vi "Stop Core.vi"(10 "final error code":i32, 11 "DAQMan in":refnum<class "Cfg Grandmaster.lvclass">) -> (3 "DAQMan out":refnum<class "Cfg Grandmaster.lvclass">)   [LabVIEW 2018, in "Configuration Grandmaster.lvlib" / "Cfg Grandmaster.lvclass"]
doc: "(<B>Filename</B>: Actor Framework.lvlib:Actor.lvclass:Stop Core.vi)\n\nDefines what the actor does before it stops. Use the <B>final error code</B> input to determine whether the actor shut down in response to an error.\n\nBy default, this method does nothing. A descendant class may override it to define behavior, such as shutting down any processes the actor initiated in its override of the Actor Core method."
uses:
  Cfg Grandmaster.lvclass
  Cfg Grandmaster.lvclass/Cfg Grandmaster.ctl
  <vilib>/ActorFramework/Stop Msg/Stop Msg.lvclass/Stop Msg.ctl
  <vilib>/ActorFramework/Message Enqueuer/Message Enqueuer.lvclass/Message Enqueuer.ctl
  <vilib>/ActorFramework/Stop Msg/Send Emergency Stop.vi
  <vilib>/ActorFramework/Stop Msg/Send Normal Stop.vi
  <vilib>/ActorFramework/Message Enqueuer/Enqueue Critical.vi
  <vilib>/ActorFramework/Message Enqueuer/Enqueue.vi
  <vilib>/ActorFramework/Stop Msg/Stop Msg.lvclass
  C:/Program Files (x86)/National Instruments/LabVIEW 2018/vi.lib/ActorFramework/Message/Message.lvclass
  <vilib>/ActorFramework/Message Priority Queue/Priority Enqueue.vi
  Actor Nest/Class Actor Nest/Actor Nest.lvclass
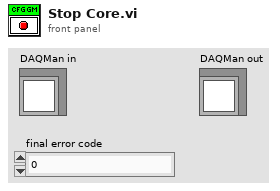
[diagram p1: front panel]
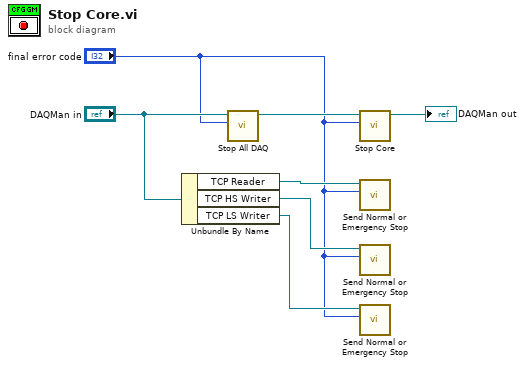
[diagram p0: block diagram]
diagram:
  n1 = Unbundle By Name("DAQMan in") -> ("TCP Reader"=w6:refnum<class "Message Enqueuer.lvclass">, "TCP HS Writer"=w5:refnum<class "Message Enqueuer.lvclass">, "TCP LS Writer"=w4:refnum<class "Message Enqueuer.lvclass">)
  n2 = call "Stop All DAQ.vi"("final error code"="final error code", "Cfg Grandmaster in"="DAQMan in") -> ("Cfg Grandmaster out"=w2:refnum<class "Cfg Grandmaster.lvclass">)  [unwired: 8 in, 1 out]
  n3 = call-parent "Stop Core.vi"("final error code"="final error code", "Actor Nest in"=w2) -> ("Actor Nest out"=→"DAQMan out":refnum<class "Cfg Grandmaster.lvclass">)  [unwired: 9 in]
  n4 = call <vilib>:"Send Normal or Emergency Stop.vi"("final error code"="final error code", "Message Enqueuer"=w6) -> ()  [unwired: 9 in, 1 out]
  n5 = call <vilib>:"Send Normal or Emergency Stop.vi"("final error code"="final error code", "Message Enqueuer"=w5) -> ()  [unwired: 9 in, 1 out]
  n6 = call <vilib>:"Send Normal or Emergency Stop.vi"("final error code"="final error code", "Message Enqueuer"=w4) -> ()  [unwired: 9 in, 1 out]
